vi "L11.vi"() -> ()   [LabVIEW 2014]
panel:
  in  "L11":dbl
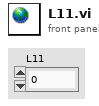
[diagram p1: front panel]
diagram:
